vi "Last Tone Played.vi"(0 "GEA2 Reference In":refnum<k24>, 5 "Standalone?":bool, 7 "Expected Tone":T1, 11 "Error In":errorcluster) -> (4 "GEA2 Reference Out":refnum<k24>, 6 "Pass/Fail?":bool, 8 "Actual Tone":T1, 15 "Error Out":errorcluster)   [LabVIEW 2014]
uses:
  type defs/Tones.ctl
  Common/LabVIEW GEA2 Toolkit/LabVIEW_GEA2_Toolkit.lvlibp/type defs/Source_Destination.ctl
  Common/LabVIEW GEA2 Toolkit/LabVIEW_GEA2_Toolkit.lvlibp/type defs/ERD Read Data In.ctl
  Common/LabVIEW GEA2 Toolkit/LabVIEW_GEA2_Toolkit.lvlibp/type defs/Data Type.ctl
  Common/LabVIEW GEA2 Toolkit/LabVIEW_GEA2_Toolkit.lvlibp
  C:/Automation/DLLs/PC Tools .NET/GeaCommunication.dll
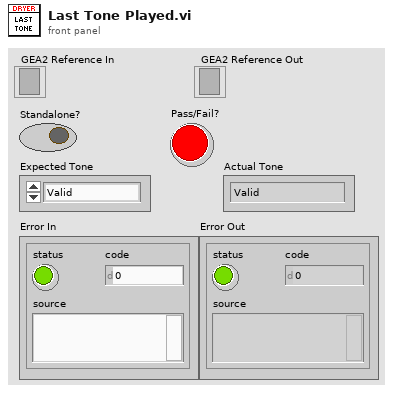
[diagram p1: front panel]
types:
  T1 = typedef "Tones.ctl" = enum16{"Valid", "Invalid", "Powerup", "Power Down", "Feature On", "Feature Off", "Hold On ", "Hold Off", "Notify Intro", "Notify End", "EOC", "Damp Alert N2", "Ext Tumble N3", "Knob", "Signal Key", "Signal Key Hold", "Unknown"}
  T2 = typedef "LabVIEW_GEA2_Toolkit.lvlibp/ERD Read Data In.ctl" = cluster{"ERD Number":u16, "Data Type":T3}
  T3 = typedef "LabVIEW_GEA2_Toolkit.lvlibp/Data Type.ctl" = enum16{"string", "boolean", "uint8_t", "uint16_t", "uint32_t", "uint64_t", "int8_t", "int16_t", "int32_t", "int64_t"}
  T4 = typedef "LabVIEW_GEA2_Toolkit.lvlibp/Source_Destination.ctl" = cluster{"Source":u8, "Destination":u8}
  T5 = typedef "LabVIEW_GEA2_Toolkit.lvlibp/ERD Read Data Out.ctl" = cluster{"ERD Number":u16, "Data":string}
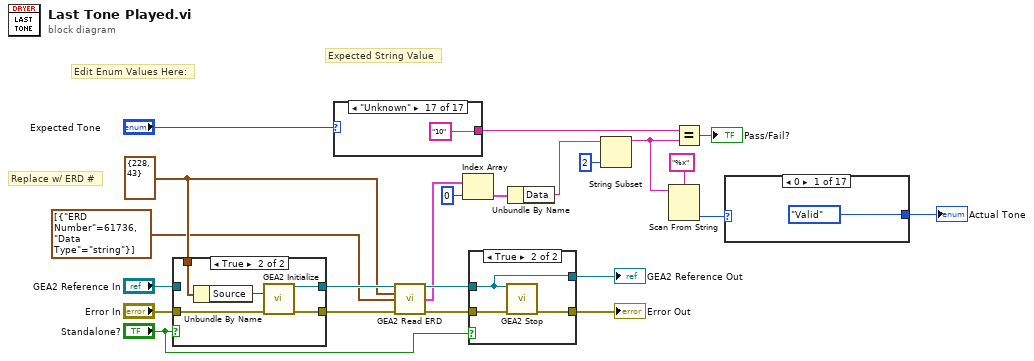
[diagram p0: block diagram]
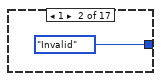
[diagram p2: hidden frame]
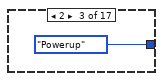
[diagram p3: hidden frame]
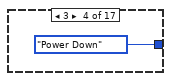
[diagram p4: hidden frame]
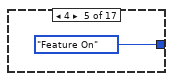
[diagram p5: hidden frame]
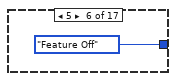
[diagram p6: hidden frame]
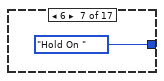
[diagram p7: hidden frame]
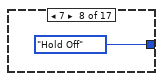
[diagram p8: hidden frame]
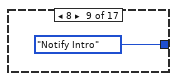
[diagram p9: hidden frame]
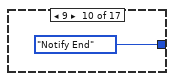
[diagram p10: hidden frame]
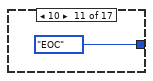
[diagram p11: hidden frame]
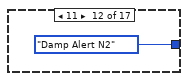
[diagram p12: hidden frame]
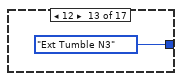
[diagram p13: hidden frame]
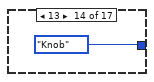
[diagram p14: hidden frame]
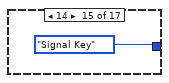
[diagram p15: hidden frame]
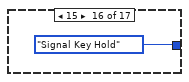
[diagram p16: hidden frame]
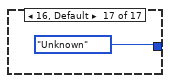
[diagram p17: hidden frame]
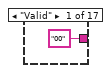
[diagram p18: hidden frame]
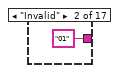
[diagram p19: hidden frame]
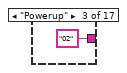
[diagram p20: hidden frame]
diagram:
  w15 = T4 {"Source"=228, "Destination"=43} ("GEA Inputs")
  # "Expected String Value"
  # "Edit Enum Values Here:"
  # "Replace w/ ERD #"
  n1 = case shown="True" "Standalone?" {
    tunnel: "Error In" -> [w24 w30]
    tunnel: [w24 w29] -> w19
    tunnel: "GEA2 Reference In" -> [w25 _]
    tunnel: [w25 w28] -> w17
    tunnel: w15 -> [_ w26]
    frame False {
    }
    frame True {
      n2 = Unbundle By Name(w26) -> ("Source"=w27:u8)
      n3 = call "GEA2 Initialize.vi"("Source Address"=w27, "error in"=w30) -> ("GEA2 Reference Out"=w28:refnum<k24>, "error out"=w29:errorcluster)  [unwired: 11 in, 1 out]
    }
  }
  n4 = case shown="\"Unknown\"" "Expected Tone" {
    tunnel: ["00" "01" "02" "03" "04" "05" "06" "07" "08" "09" "0A" "0B" "0C" "0D" "0E" "0F" "10"] -> w8
    frame "Valid" {
    }
    frame "Invalid" {
    }
    frame "Powerup" {
    }
    frame "Power Down" {
    }
    frame "Feature On" {
    }
    frame "Feature Off" {
    }
    frame "Hold On " {
    }
    frame "Hold Off" {
    }
    frame "Notify Intro" {
    }
    frame "Notify End" {
    }
    frame "EOC" {
    }
    frame "Damp Alert N2" {
    }
    frame "Ext Tumble N3" {
    }
    frame "Knob" {
    }
    frame "Signal Key" {
    }
    frame "Signal Key Hold" {
    }
    frame "Unknown" {
    }
  }
  n5 = call "GEA2 Read ERD.vi"("GEA2 Reference In"=w17, "GEA Inputs"=w15, "Read ERD List"=T2[] [{"ERD Number"=61736, "Data Type"=enum."string"}], "Error In"=w19) -> ("GEA2 Reference Out"=w16:refnum<k24>, "ERD Data Out"=w13:T5[], "Error Out"=w18:errorcluster)  [unwired: 8 in, 1 out]
  n6 = Index Array(array=w13, index=0) -> (element=w11:T5)
  n7 = case shown="True" "Standalone?" {
    tunnel: [w49 w52] -> w21
    tunnel: w18 -> [w49 w51]
    tunnel: w16 -> [w48 w50]
    tunnel: [w48 w50] -> w5
    frame False {
    }
    frame True {
      n8 = call "GEA2 Stop.vi"("GEA2 Reference In"=w50, "Error In"=w51) -> ("Error Out"=w52:errorcluster)  [unwired: 13 in]
    }
  }
  "Error Out" <- w21
  "GEA2 Reference Out" <- w5
  n9 = Unbundle By Name(w11) -> ("Data"=w10:string)
  n10 = String Subset(string=w10, length (rest)=2 ("length (rest)")) -> (substring=w4:string)  [unwired: 1 in]
  n11 = Scan From String(format string="%x", input string=w4) -> (output 1=w2:u32)  [unwired: 3 in, 3 out]
  n12 = Equal?(x=w8, y=w4) -> (x = y?=→"Pass/Fail?":bool)
  n13 = case shown="0" w2 {
    tunnel: [Tones."Valid" ("Expected Tone 2") Tones."Invalid" ("Expected Tone 2") Tones."Powerup" ("Expected Tone 2") Tones."Power Down" ("Expected Tone 2") Tones."Feature On" ("Expected Tone 2") Tones."Feature Off" ("Expected Tone 2") Tones."Hold On " ("Expected Tone 2") Tones."Hold Off" ("Expected Tone 2") Tones."Notify Intro" ("Expected Tone 2") Tones."Notify End" ("Expected Tone 2") Tones."EOC" ("Expected Tone 2") Tones."Damp Alert N2" ("Expected Tone 2") Tones."Ext Tumble N3" ("Expected Tone 2") Tones."Knob" ("Expected Tone 2") Tones."Signal Key" ("Expected Tone 2") Tones."Signal Key Hold" ("Expected Tone 2") Tones."Unknown" ("Expected Tone 2")] -> w1
    frame 0 {
    }
    frame 1 {
    }
    frame 2 {
    }
    frame 3 {
    }
    frame 4 {
    }
    frame 5 {
    }
    frame 6 {
    }
    frame 7 {
    }
    frame 8 {
    }
    frame 9 {
    }
    frame 10 {
    }
    frame 11 {
    }
    frame 12 {
    }
    frame 13 {
    }
    frame 14 {
    }
    frame 15 {
    }
    frame 16, Default {
    }
  }
  "Actual Tone" <- w1
